vi "usb capture req only.vi"() -> (3 "function return":bool)   [LabVIEW 2018, in "Dll1_x64_191014_0.lvlib"]
doc: "__declspec(dllexport) bool usb_capture_req_only();"
uses:
  <userlib>/Dll1_x64_191014_0/Dll1_x64_191014_0.lvlib
  <userlib>/Dll1_x64_191014_0/Dll1.dll
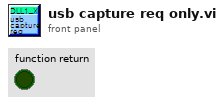
[diagram p1: front panel]
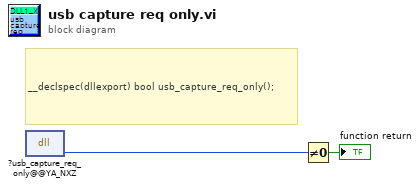
[diagram p0: block diagram]
diagram:
  # "__declspec(dllexport) bool usb_capture_req_only();"
  n1 = dll-call lib="C:/Program Files/National Instruments/LabVIEW 2018/user.lib/Dll1_x64_191014_0/Dll1.*" fn="?usb_capture_req_only@@YA_NXZ"() -> (w1:u8)  [unwired: 3 in, 2 out]
  n2 = Not Equal To 0?(x=w1) -> (x != 0?=→"function return":bool)
